vi "Get Variable.vi"(8 "error in (no error)":errorcluster, 10 "Name":string, 11 "Project in":refnum<class "Project.lvclass">) -> (0 "error out":errorcluster, 2 "Value":variant, 3 "Project out":refnum<class "Project.lvclass">)   [LabVIEW 2015, in "Project.lvclass"]
uses:
  Project.lvclass
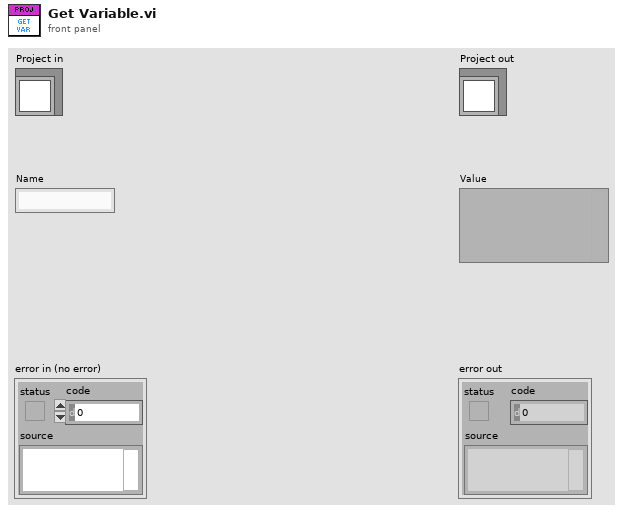
[diagram p1: front panel]
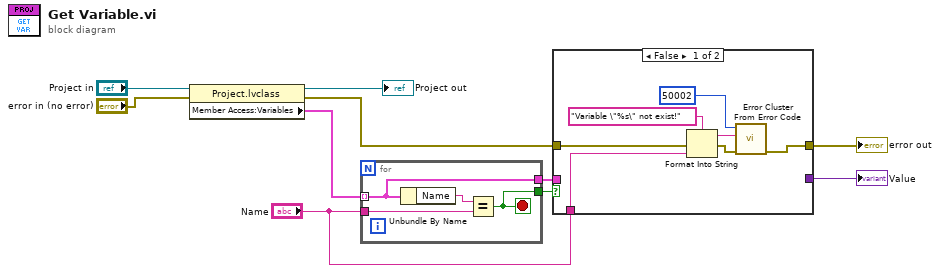
[diagram p0: block diagram]
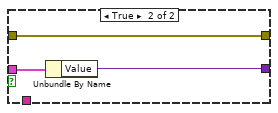
[diagram p2: hidden frame]
diagram:
  n1 = property class="Project.lvclass"(reference="Project in", error in="error in (no error)") -> (reference out=→"Project out":refnum<class "Project.lvclass">, error out=w3:errorcluster, "Member Access:Variables"=w10:cluster{"Name":string, "Value":variant}[])
  n2 = for {
    tunnel: "Name" -> [w13]
    tunnel: w10 -> [w12] mode=indexing
    tunnel: [w12] -> w9
    tunnel: [w11] -> w4
    stop <- w11 stop-if-true
    n3 = Unbundle By Name(w12) -> ("Name"=w14:string)
    n4 = Equal?(x=w14, y=w13) -> (x = y?=w11:bool)
  }
  n5 = case shown="False" w4 {
    tunnel: w9 -> [_ w24]
    tunnel: [_ w23] -> w5
    tunnel: w3 -> [w20 w22]
    tunnel: "Name" -> [w19 _]
    tunnel: [w16 w22] -> w1
    frame False {
      n6 = Format Into String(format string="Variable \"%s\" not exist!" ("error message (\"\")"), error in=w20, w19) -> (resulting string=w18:string, error out=w17:errorcluster)  [unwired: 1 in]
      n7 = call <vilib>:"Error Cluster From Error Code.vi"("error in (no error)"=w17, "error message (\"\")"=w18, "error code (0)"=50002) -> ("error out"=w16:errorcluster)  [unwired: 6 in]
    }
    frame True {
      n8 = Unbundle By Name(w24) -> ("Value"=w23:variant)
    }
  }
  "error out" <- w1
  "Value" <- w5
